vi "Create with Type Override.vi"(6 "Type Override":string, 7 "Direction":T1, 8 "error in (no error)":errorcluster, 9 "Custom Config Data":u8[](array[numeric]), 10 "Name":string, 11 "CIFFIFO in":refnum<class "CIF_CIPC_Fifo_U8.lvclass">) -> (0 "error out":errorcluster, 3 "CIFFIFO out":refnum<class "CIF_CIPC_Fifo_U8.lvclass">)   [LabVIEW 2021, in "CIF_CIPC_Fifo_U8.lvclass"]
uses:
  CIF_CIPC_Fifo_U8.lvclass
  CIF_CIPC_Fifo_U8.lvclass/CIF_CIPC_Fifo_U8.ctl
  CIFChannels/Typedef/Direction.ctl
  CIFChannels/CIFChannels.lvclass
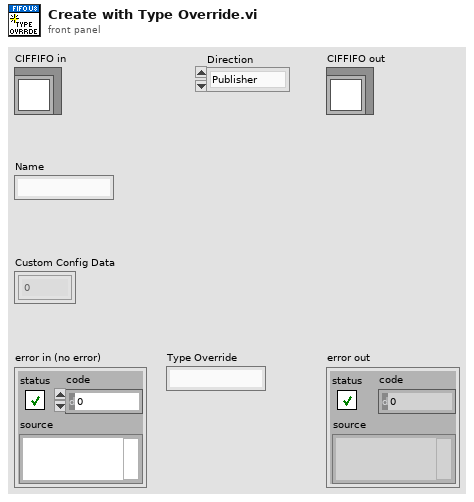
[diagram p1: front panel]
types:
  T1 = typedef "CIFChannels.lvclass/Direction.ctl" = enum16{"Publisher", "Subscriber"}
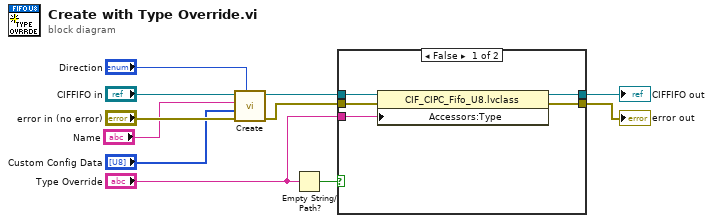
[diagram p0: block diagram]
diagram:
  n1 = call-dynamic "Create.vi"("Direction"="Direction", "error in (no error)"="error in (no error)", "Custom Config Data"="Custom Config Data", "Name"="Name", "CIFFIFO in"="CIFFIFO in") -> ("error out"=w5:errorcluster, "CIFFIFO out"=w6:refnum<class "CIF_CIPC_Fifo_U8.lvclass">)  [unwired: 5 in]
  n2 = Empty String/Path?(string/path="Type Override") -> (empty?=w3:bool)
  n3 = case shown="False" w3 {
    tunnel: w6 -> [w16 w18]
    tunnel: "Type Override" -> [w15 _]
    tunnel: w5 -> [w14 w17]
    tunnel: [w13 w18] -> w2
    tunnel: [w12 w17] -> w1
    frame False {
      n4 = property class="CIF_CIPC_Fifo_U8.lvclass"(reference=w16, error in=w14, "Accessors:Type"=w15) -> (reference out=w13:refnum<class "CIF_CIPC_Fifo_U8.lvclass">, error out=w12:errorcluster)
    }
    frame True {
    }
  }
  "error out" <- w1
  "CIFFIFO out" <- w2
